vi "Core Write U8 FIFO.vi"(8 "error in (no error)":errorcluster, 9 "Timeout (ms)":i32, 10 "U8 With Header in":u8[](array[numeric]), 11 "CIFFIFO in":refnum<class "CIF_NIChn_Fifo_U8.lvclass">) -> (0 "error out":errorcluster, 1 "timed out?":bool, 2 "U8 With Header out":u8[](array[numeric]), 3 "CIFFIFO out":refnum<class "CIF_NIChn_Fifo_U8.lvclass">)   [LabVIEW 2021, in "CIF_NIChn_Fifo_U8.lvclass"]
uses:
  CIF_NIChn_Fifo_U8.lvclass
  CIF_NIChn_Fifo_U8.lvclass/CIF_NIChn_Fifo_U8.ctl
  NIChn/CIF_NIChn.lvclass
  <vilib>/CIF Foundation/NI Channels/NIChannels.lvlib
  CIFChannels/CIFChannels.lvclass
  1bad10da-a98b-49ee-b03a-18b497e396df.vi
  70f860b1-5d4a-43dc-b0c2-c9446e8447f7.vi
  D:/dev/Packages/Channel_Manager/src/CIFChannels/CIFChannels.lvclass
  D:/dev/Packages/Channel_Manager/src/CIF_NIChn/NIChn/CIF_NIChn.lvclass
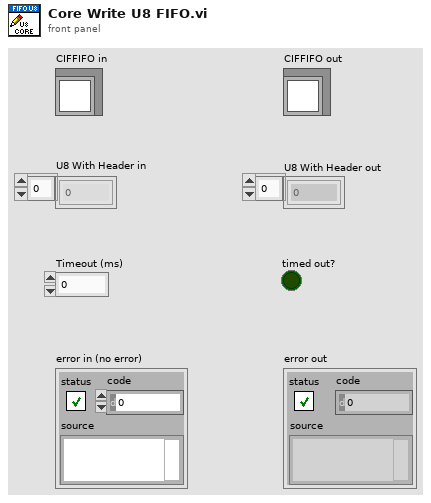
[diagram p1: front panel]
types:
  T1 = typedef "ChannelCommon.lvlib/FIFO Header.ctl" = cluster{"Length":u64, "T0":i64, "T_Out":i64, "T_Tx":i64, "Ctr":u64, "ClockID":u8}
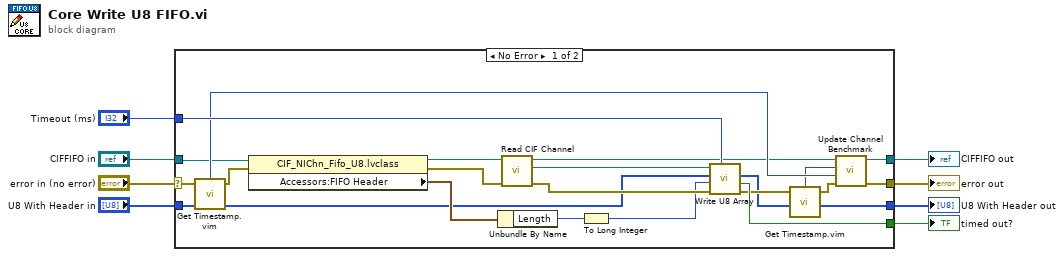
[diagram p0: block diagram]
diagram:
  n1 = case shown="No Error" "error in (no error)" {
    selector: "error in (no error)" -> [w14 w32]
    tunnel: [w22 w32] -> w7
    tunnel: [w21 w31] -> w2
    tunnel: "CIFFIFO in" -> [w16 w31]
    tunnel: [w29 _] -> w6
    tunnel: "Timeout (ms)" -> [w28 _]
    tunnel: "U8 With Header in" -> [w17 w30]
    tunnel: [w9 w30] -> w1
    frame No Error {
      n2 = call "Get Timestamp.vim"("Anything in"=w14) -> ("Time (ns)"=w20:i64, "Anything out"=w13:errorcluster)  [unwired: 2 in]
      n3 = property class="CIF_NIChn_Fifo_U8.lvclass"(reference=w16, error in=w13) -> (reference out=w18:refnum<class "CIF_NIChn_Fifo_U8.lvclass">, error out=w23:errorcluster, "Accessors:FIFO Header"=w25:T1)
      n4 = Unbundle By Name(w25) -> ("Length"=w24:u64)
      n5 = call "Read CIF Channel.vi"("error in (no error)"=w23, "CIFTag in"=w18) -> ("error out"=w27:errorcluster, "CIF Channel"=w26:refnum<k21>, "CIFTag out"=w15:refnum<class "CIF_NIChn_Fifo_U8.lvclass">)  [unwired: 7 in]
      n6 = To Long Integer(number=w24) -> (32bit integer=w10:i32)
      n7 = call <vilib>:"Write U8 Array.vi"("Timeout (ms)"=w28, "error in"=w27, "Number of Elements"=w10, "U8 Array in"=w17, "CIF Channel in"=w26) -> ("error out"=w12:errorcluster, "Timed out?"=w29:bool, "U8 Array out"=w9:u8[])  [unwired: 3 in, 1 out]
      n8 = call "Get Timestamp.vim"("Anything in"=w12) -> ("Time (ns)"=w19:i64, "Anything out"=w11:errorcluster)  [unwired: 2 in]
      n9 = call "Update Channel Benchmark.vi"("error in (no error)"=w11, "X0"=w20, "X1"=w19, "CIFChannels in"=w15) -> ("error out"=w22:errorcluster, "CIFChannels out"=w21:refnum<class "CIF_NIChn_Fifo_U8.lvclass">)  [unwired: 6 in]
    }
    frame Error {
    }
  }
  "error out" <- w7
  "CIFFIFO out" <- w2
  "timed out?" <- w6
  "U8 With Header out" <- w1
